vi "TDS 2004B Two Channel Initialize SubVI.vi"(0 "VISA resource name":refnum<visa-resource-name>, 1 "Channel A":i32(ring) items=["Channel 1", "Channel 2", "Channel 3", "Channel 4", "Math", "Reference A", "Reference B", "Reference C", "Reference D"], 4 "Ch A Vertical Range (10.0 V/div)":dbl=10.0, 5 "Ch A Vertical Offset (0.0 divs)":dbl, 6 "Timebase (0.0005 s)":dbl=0.0005, 7 "error in (no error)":errorcluster, 8 "Serial Configuration":T1={"Baud Rate"=19200, "Parity"=0, "Stop Bits"=10, "Flow Control"=2} {"Flow Control" items=["None", "XON/XOFF", "RTS/CTS", "XON/XOFF & RTS/CTS", "DTR/DSR", "XON/XOFF & DTR/DSR"]; "Stop Bits" items=["1.0"=10, "1.5"=15, "2.0"=20]; "Parity" items=["None", "Odd", "Even", "Mark", "Space"]; "Baud Rate" items=["300"=300, "600"=600, "1200"=1200, "2400"=2400, "4800"=4800, "9600"=9600, "19200"=19200]}, 9 "Trigger Level (0.0 V)":dbl=1.0, 10 "Acquisition Type (0: Sample)":i32(ring) items=["Sample", "Average", "Peak Detect"], 11 "Number of Averaged Waveforms (4: 4)":i32(ring)=4 items=["4"=4, "16"=16, "64"=64, "128"=128], 12 "Position (0.0 s)":dbl, 15 "Channel B":i32(ring)=1 items=["Channel 1", "Channel 2", "Channel 3", "Channel 4", "Math", "Reference A", "Reference B", "Reference C", "Reference D"], 17 "Trigger Slope (0: Rising)":i32(ring) items=["Rising", "Falling"], 18 "Ch B Vertical Range (10.0 V/div)":dbl=10.0, 19 "Ch B Vertical Offset (0.0 divs)":dbl) -> (13 "error out":errorcluster, 14 "VISA resource name out":refnum<visa-resource-name>)   [LabVIEW 2017]
uses:
  Program Files/National Instruments/LabVIEW 2017/instr.lib/Tektronix TDS 200 1000 2000 Series/Tektronix TDS 200 1000 2000 Series.lvlib
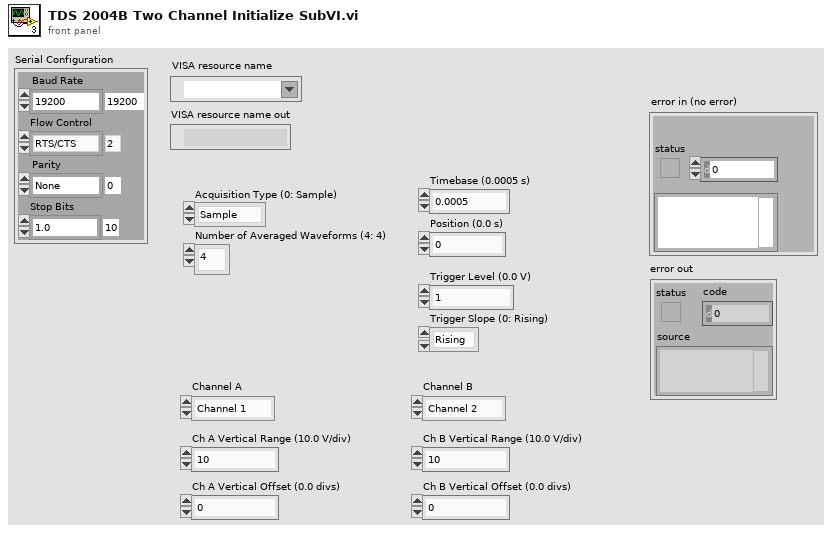
[diagram p1: front panel]
types:
  T1 = cluster{"Baud Rate":u32, "Parity":u16, "Stop Bits":u16, "Flow Control":u16}
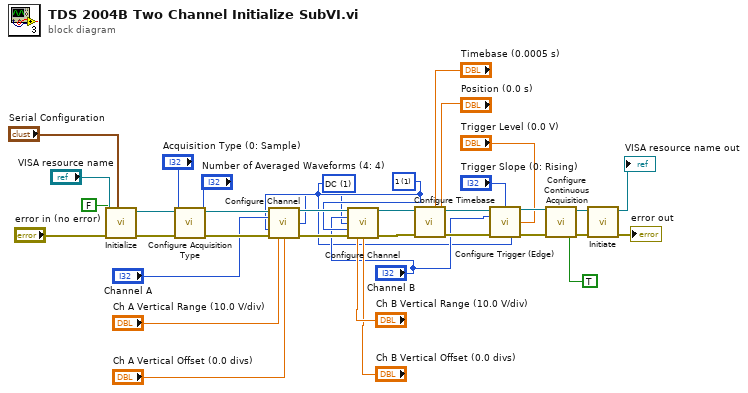
[diagram p0: block diagram]
diagram:
  w17 = 1 items=["1"=1, "10"=10, "20"=20, "50"=50, "100"=100, "500"=500, "1000"=1000] ("Probe Attenuation (10: 10X)")
  w3 = 1 items=["AC", "DC", "Ground"] ("Vertical Coupling (1: DC)")
  n1 = call "Initialize.vi"("Serial Configuration"="Serial Configuration", "error in (no error)"="error in (no error)", "Reset? (T: Yes)"=FALSE, "VISA resource name"="VISA resource name") -> ("error out"=w25:errorcluster, "VISA resource name out"=w23:refnum<visa-resource-name>)  [unwired: 6 in]
  n2 = call "Configure Acquisition Type.vi"("error in (no error)"=w25, "Number of Averaged Waveforms (4: 4)"="Number of Averaged Waveforms (4: 4)", "Acquisition Type (0: Sample)"="Acquisition Type (0: Sample)", "VISA resource name"=w23) -> ("error out"=w24:errorcluster, "VISA resource name out"=w22:refnum<visa-resource-name>)  [unwired: 6 in]
  n3 = call "Configure Channel.vi"("VISA resource name"=w22, "Channel (0: Channel 1)"="Channel A", "Vertical Coupling (1: DC)"=w3, "Probe Attenuation (10: 10X)"=w17, "error in (no error)"=w24, "Vertical Range (10.0 V/div)"="Ch A Vertical Range (10.0 V/div)", "Vertical Offset (0.0 divs)"="Ch A Vertical Offset (0.0 divs)") -> ("VISA resource name out"=w32:refnum<visa-resource-name>, "error out"=w33:errorcluster)  [unwired: 7 in]
  n4 = call "Configure Channel.vi"("VISA resource name"=w32, "Channel (0: Channel 1)"="Channel B", "Vertical Coupling (1: DC)"=w3, "Probe Attenuation (10: 10X)"=w17, "error in (no error)"=w33, "Vertical Range (10.0 V/div)"="Ch B Vertical Range (10.0 V/div)", "Vertical Offset (0.0 divs)"="Ch B Vertical Offset (0.0 divs)") -> ("VISA resource name out"=w35:refnum<visa-resource-name>, "error out"=w34:errorcluster)  [unwired: 7 in]
  n5 = call "Configure Timebase.vi"("error in (no error)"=w34, "Position (0.0 s)"="Position (0.0 s)", "Timebase (0.0005 s)"="Timebase (0.0005 s)", "VISA resource name"=w35) -> ("error out"=w27:errorcluster, "VISA resource name out"=w26:refnum<visa-resource-name>)  [unwired: 6 in]
  n6 = call "Configure Trigger (Edge).vi"("VISA resource name"=w26, "Trigger Source (0: Channel 1)"="Channel B", "Trigger Level (0.0 V)"="Trigger Level (0.0 V)", "error in (no error)"=w27, "Trigger Slope (0: Rising)"="Trigger Slope (0: Rising)", "Trigger Coupling (0: AC)"=w3) -> ("VISA resource name out"=w28:refnum<visa-resource-name>, "error out"=w29:errorcluster)  [unwired: 8 in]
  n7 = call "Configure Continuous Acquisition.vi"("error in (no error)"=w29, "Enable Continuous Acquisition Mode (True)"=TRUE, "VISA resource name"=w28) -> ("error out"=w31:errorcluster, "VISA resource name out"=w30:refnum<visa-resource-name>)  [unwired: 7 in]
  n8 = call "Initiate.vi"("error in (no error)"=w31, "VISA resource name"=w30) -> ("error out"=→"error out":errorcluster, "VISA resource name out"=→"VISA resource name out":refnum<visa-resource-name>)  [unwired: 8 in]
